vi "Init.vi"(8 "error in (no error)":errorcluster, 9 "Config File Path":path=path "", 10 "Name":string, 11 "Mock Error Handler In":refnum<class "Mock Error Handler.lvclass">) -> (0 "error out":errorcluster, 3 "Mock Error Handler Out":refnum<class "Mock Error Handler.lvclass">)   [LabVIEW 2020, in "Mock Error Handler.lvclass"]
doc: "Initializes the process and creates necessary references. Anything initialized here is released in the Clear.vi method."
uses:
  Mock Error Handler.lvclass
  Private/Error Message Data.ctl
  Mock Error Handler.lvclass/Mock Error Handler.ctl
  Framework/Process/Process.lvclass
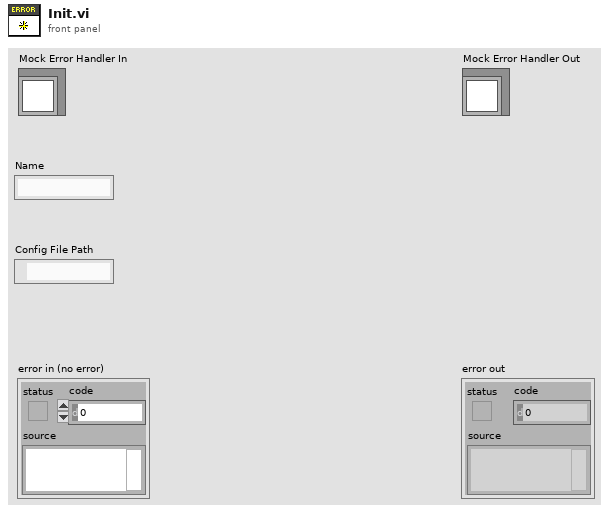
[diagram p1: front panel]
types:
  T1 = typedef "Mock Error Handler.lvclass/Error Message Data.ctl" = cluster{"Location":string, "Error":errorcluster}
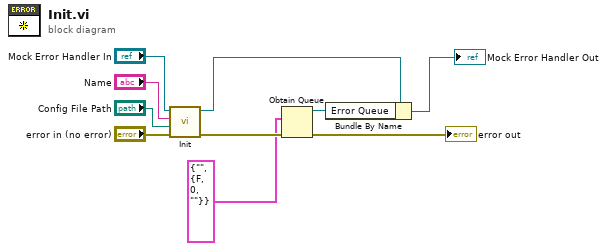
[diagram p0: block diagram]
diagram:
  n1 = call-parent "Init.vi"("error in (no error)"="error in (no error)", "Config File Path"="Config File Path", "Name"="Name", "Process In"="Mock Error Handler In") -> ("error out"=w3:errorcluster, "Process Out"=w6:refnum<class "Mock Error Handler.lvclass">)  [unwired: 6 in]
  n2 = Obtain Queue(element data type=T1 {"Location"="", "Error"={"status"=FALSE, "code"=0, "source"=""}} ("Error Message Data"), error in (no error)=w3) -> (queue out=w1:refnum<queue>, error out=→"error out":errorcluster)  [unwired: 3 in, 1 out]
  n3 = Bundle By Name(cluster=w6, "Error Queue"=w1) -> (→"Mock Error Handler Out":refnum<class "Mock Error Handler.lvclass">)
